vi "Get Index Set.vi"(8 "error in (no error)":errorcluster, 9 "Expected Type":T1, 11 "Tag Names":string[](array[string])) -> (0 "error out":errorcluster, 3 "Tag References":i32[](array[numeric]))   [LabVIEW 2010, in "Current Value Table.lvlib"]
doc: "This VI retrieves a group of indices as defined by the tag names provided. These tags must be retrieved as a single type. If multiple types are requested, error 537165 will be thrown."
uses:
  Current Value Table.lvlib
  Type Defs/Data Types.ctl
  FGVs/Tag Memory Methods.ctl
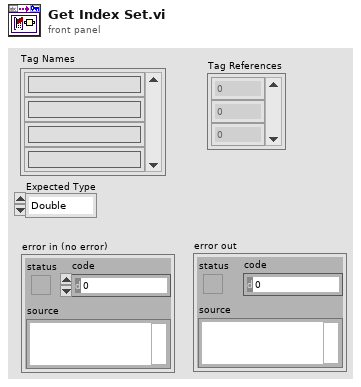
[diagram p1: front panel]
types:
  T1 = typedef "Current Value Table.lvlib/Data Types.ctl" = enum16{"Double", "Single", "I64", "I32", "I16", "I8", "U64", "U32", "U16", "U8", "String", "Boolean", "Array of U8", "Array of U16", "Array of U32", "Array of U64", "Array of I64", "Array of I32", "Array of I16", "Array of I8", "Array of Double", "Array of Single", "Array of Boolean", "Array of String"}
  T2 = typedef "Current Value Table.lvlib/Tag Memory Methods.ctl" = enum16{"Clear", "Read Tag Index", "Read Tag Indices", "Generate Group", "Add Tag", "Overwrite Tag", "Read Description", "Get Stored Tags"}
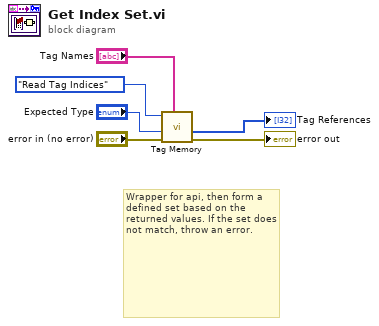
[diagram p0: block diagram]
diagram:
  # "Wrapper for api, then form a defined set based on the returned values. If the set does not match, throw an error."
  n1 = call "Tag Memory.vi"("Tags"="Tag Names", "error in (no error)"="error in (no error)", "Expected Type"="Expected Type", "Method"=Tag_Memory_Methods."Read Tag Indices") -> ("error out"=→"error out":errorcluster, "Indices Out"=→"Tag References":i32[])  [unwired: 2 in, 4 out]
